vi "tb_interp_fft_fpga.vi"() -> ()   [LabVIEW 2011]
uses:
  <vilib>/Platform/TimedLoop/XDataNode/XDataNode.xnode
  <vilib>/Platform/TimedLoop/XDataNode/nitl_modes.ctl
  <vilib>/Platform/TimedLoop/XDataNode/XDNodeRunTimeDep.lvlib
  <vilib>/Platform/TimedLoop/XDataNode/wakeup.ctl
  <vilib>/Platform/TimedLoop/XDataNode/timing_clust.ctl
  <vilib>/rvi/DataTransferAndStorage/Container/XNode/niFpgaContainer.xnode
  <vilib>/rvi/FXPMathLib/FxpInterpret/XNode/nifxpmath_Interpret.xnode
  <userlib>/FPGA Library/Code Development/Signal Processing/Interpolation Block/Controls/Interpolation Input Data.ctl
  <vilib>/eio/EIONode/EIONode.xnode
  <vilib>/rvi/FIFO/Fifo_Resource/nirvififoEmulationGetNumberOfElementsToRead.vi
  <vilib>/rvi/FIFO/Fifo_Resource/nirvififoEmulationRead.vi
  <vilib>/rvi/interface/RandomDataEmulation/nirviRandomDataFpgaReadWriteTemplate.vi
  <vilib>/rvi/FIFO/Fifo_Resource/nirvififoEmulationWrite.vi
  <vilib>/rvi/eio/common/nirviEmuTemplateMethod_errors.vi
  <userlib>/FPGA Library/Code Development/Signal Processing/FFT Block/FFT/Controls/FFT States.ctl
  <userlib>/FPGA Library/Code Development/Signal Processing/FFT Block/FFT/Controls/FFT Parameters.ctl
panel:
  in  "FFT Parameters":T1={"Direction"=TRUE, "scale_sch"=85.0, "Flush Length"=0} {"scale_sch" format="%.0b"}
  in  "FFT State":cluster{"FFT State":T2, "Set FFT State?":bool}
  out "acq timed out?":bool
  out "Numeric":i32
  out "Interp Loop Overflow":bool
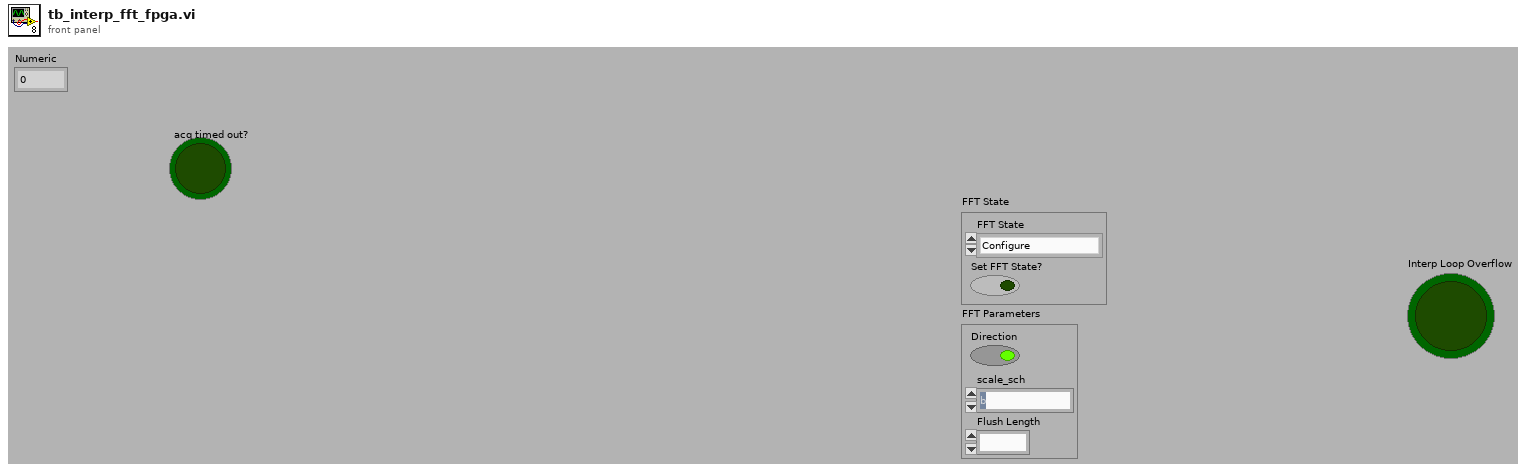
[diagram p1: front panel]
types:
  T1 = typedef "FFT Parameters.ctl" = cluster{"Direction":bool, "scale_sch":fxp<+,10,10>, "Flush Length":u16}
  T2 = typedef "FFT States.ctl" = enum8{"Configure", "Start FFT processing", "Process", "Unload Last FFT", "Reset"}
  T3 = typedef "XDNodeRunTimeDep.lvlib/timing_clust.ctl" = cluster{"Expected End [f-1]":u64, "Actual End [f-1]":u64, "Finished Late? [f-1]":bool, "Expected End [i-1]":u64, "Actual End [i-1]":u64, "Finished Late? [i-1]":bool, "Expected Start [i]":u64, "Actual Start [i]":u64, "Expected Start [f]":u64, "Actual Start [f]":u64, "Source Name":string, "Structure Name":string, "Period":i64, "Deadline":i64, "Offset":i64, "Start":i64, "Priority":i32, "Timeout":i32, "Mode":T4, "Wakeup Reason":T5, "Error":errorcluster, "Source Type":string, "Secondary Source Type":string, "Global End Time":u64, "Global Start Time":u64, "Frame Duration":u64, "Iteration Duration":u64, "Assigned CPU":i32, "I/O Scan Engine Mode":u32}
  T4 = typedef "XDNodeRunTimeDep.lvlib/nitl_modes.ctl" = enum32{"No Change", "Process missed periods, maintain original phase", "Discard missed periods, maintain original phase", "Process missed periods, ignore original phase", "Discard missed periods, ignore original phase"}
  T5 = typedef "XDNodeRunTimeDep.lvlib/wakeup.ctl" = enum32{"Normal", "Aborted", "Asynchronous wakeup", "Timing source error", "Timed loop error", "Timeout"}
  T6 = typedef "Interpolation Input Data.ctl" = fxp<+/-,18,1>
  T7 = typedef "Interpolation Output Data.ctl" = fxp<+/-,19,1>
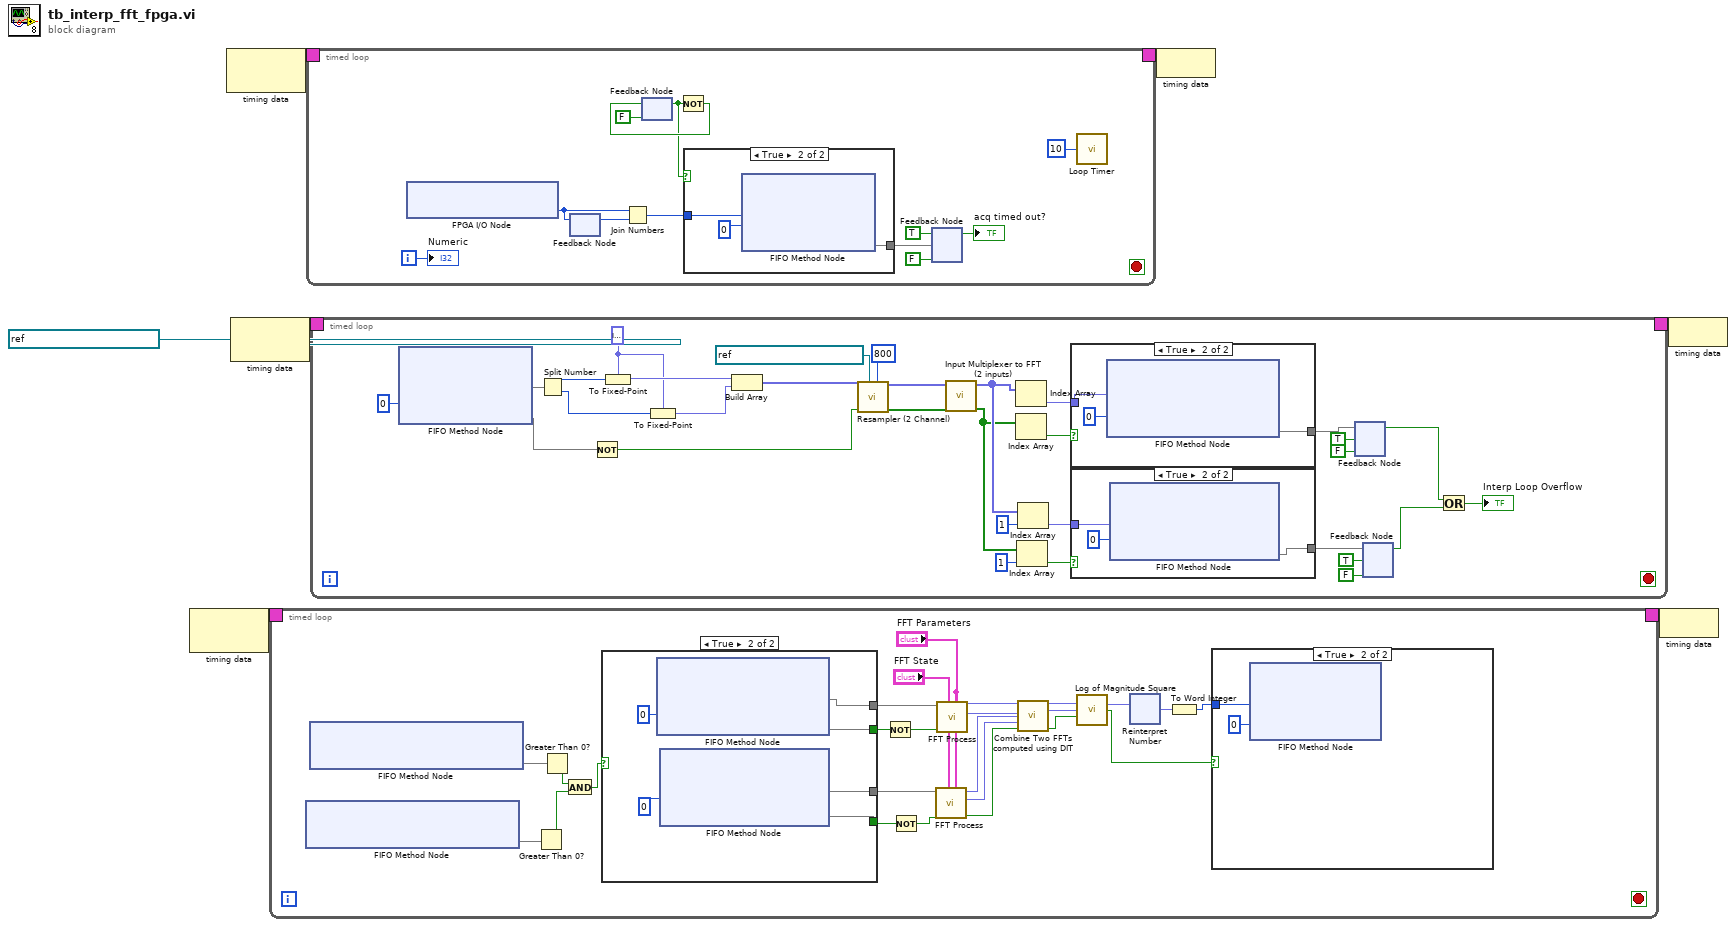
[diagram p0: block diagram]
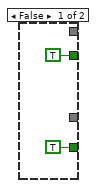
[diagram p4: hidden frame]
diagram:
  n1 = node-c288() -> (w5:T3)  [unwired: 1 in]
  n2 = node-c288() -> (w2:T3)  [unwired: 1 in]
  n3 = node-c288(refnum<k21> "40 MHz Onboard Clock" ("Source Name")) -> (w7:T3)
  n4 = timed-loop {
    timing: w5 -> [_]
    timing-out: [_] -> w4
    stop <- _ stop-if-true
    n5 = xnode ("FIFO Method Node")() -> ("Number of Elements to Read"=w24)  [unwired: 1 in, 1 out]
    n6 = xnode ("FIFO Method Node")() -> ("Number of Elements to Read"=w25)  [unwired: 1 in, 1 out]
    n7 = Greater Than 0?(x=w24) -> (x > 0?=w22:bool)
    n8 = Greater Than 0?(x=w25) -> (x > 0?=w23:bool)
    n9 = And(x=w23, y=w22) -> (x .and. y?=w21:bool)
    n10 = case shown="True" w21 {
      tunnel: [TRUE ("Timed Out?") w40] -> w32
      tunnel: [_ w39] -> w31
      tunnel: [_ w38] -> w30
      tunnel: [TRUE ("Timed Out?") w37] -> w29
      frame False {
      }
      frame True {
        n11 = xnode ("FIFO Method Node")("Timeout"=0) -> ("Element"=w39, "Timed Out?"=w40)  [unwired: 1 in, 1 out]
        n12 = xnode ("FIFO Method Node")("Timeout"=0) -> ("Element"=w38, "Timed Out?"=w37)  [unwired: 1 in, 1 out]
      }
    }
    n13 = Not(x=w32) -> (.not. x?=w26:bool)
    n14 = Not(x=w29) -> (.not. x?=w27:bool)
    n15 = call <userlib>:"FFT Process.vi"("FFT Parameters"="FFT Parameters", "FFT State"="FFT State", "Input Valid"=w27, "Real Data In"=w30) -> ("Output Valid"=w13:bool, "Imag Data Out"=w14:fxp<+/-,16,1>, "Real Data Out"=w15:fxp<+/-,16,1>)  [unwired: 2 in, 3 out]
    n16 = call <userlib>:"FFT Process.vi"("FFT Parameters"="FFT Parameters", "FFT State"="FFT State", "Input Valid"=w26, "Real Data In"=w31) -> ("Imag Data Out"=w16:fxp<+/-,16,1>, "Real Data Out"=w17:fxp<+/-,16,1>)  [unwired: 2 in, 4 out]
    n17 = call <userlib>:"Combine Two FFTs computed using DIT.vi"("Real FFT 1"=w17, "Imag FFT 1"=w16, "Real FFT 2"=w15, "Imag FFT 2"=w14, "Input Data Valid"=w13) -> ("Real FFT k"=w12:fxp<+/-,24,3>, "Imag FFT k"=w11:fxp<+/-,24,3>, "Output Valid"=w10:bool)  [unwired: 6 in, 2 out]
    n18 = call <userlib>:"Log of Magnitude Square.vi"("Real"=w12, "Imaginary"=w11, "Input Valid"=w10) -> ("Log Magnitude"=w20:fxp<+/-,34,12>, "Output Valid"=w18:bool)  [unwired: 11 in]
    n19 = xnode "Reinterpret Number"("x"=w20) -> ("y"=w28:fxp<+/-,34,16>)
    n20 = To Word Integer(number=w28) -> (16bit integer=w19:i16)
    n21 = case shown="True" w18 {
      tunnel: w19 -> [_ w34]
      frame False {
      }
      frame True {
        n22 = xnode ("FIFO Method Node")("Element"=w34, "Timeout"=0) -> ()  [unwired: 1 in, 2 out]
      }
    }
  }
  n23 = timed-loop {
    timing: w2 -> [_]
    timing-out: [_] -> w1
    i -> [w52]
    stop <- _ stop-if-true
    n24 = xnode "FPGA I/O Node"() -> ("IO Module\\AI 0 Data"=w61:i16)  [unwired: 1 in, 1 out]
    n25 = feedback-in #1(w61) -> ()
    n26 = feedback #1() -> (w60:i16)  [unwired: 1 in]
    n27 = Join Numbers(hi=w61, lo=w60) -> ((hi.lo)=w50:u32)
    n28 = feedback #2(FALSE) -> (w51:bool)
    n29 = Not(x=w51) -> (.not. x?=w59:bool)
    n30 = feedback-in #2(w59) -> ()
    n31 = case shown="True" w51 {
      tunnel: w50 -> [_ w64]
      tunnel: [_ w62] -> w55
      frame False {
      }
      frame True {
        n32 = xnode ("FIFO Method Node")("Element"=w64, "Timeout"=0) -> ("Timed Out?"=w62)  [unwired: 1 in, 1 out]
      }
    }
    n33 = feedback-in #3(TRUE, w55) -> ()
    n34 = feedback #3(FALSE) -> (→"acq timed out?":bool)
    n35 = call "Loop Timer"("Count(mSec)"=u32 10) -> ()  [unwired: 1 out]
    "Numeric" <- w52
  }
  n36 = timed-loop {
    timing: w7 -> [_]
    timing-out: [_] -> w6
    stop <- _ stop-if-true
    w72 = T6 0.0 ("Interpolate.Input Data")
    n37 = xnode ("FIFO Method Node")("Timeout"=0) -> ("Element"=w78, "Timed Out?"=w70)  [unwired: 1 in, 1 out]
    n38 = Split Number(x=w78) -> (hi(x)=w76:u16, lo(x)=w75:u16)
    n39 = Not(x=w70) -> (.not. x?=w69:bool)
    n40 = To Fixed-Point(fixed-point type=w72, number=w76) -> (fixed-point=w73:T6)
    n41 = To Fixed-Point(fixed-point type=w72, number=w75) -> (fixed-point=w74:T6)
    n42 = Build Array(w73, w74) -> (w71:T6[])
    n43 = call <userlib>:"Resampler (2 Channel).vi"("CalibrationTable Length-1"=u16 800, "ResampleVectorInfo"=refnum<k21> "Resample Vector Table", "DataValid"=w69, "Input Data"=w71) -> ("Data Valid"=w96:bool[], "Interpolated Data"=w97:T7[])  [unwired: 6 in]
    n44 = call <userlib>:"Input Multiplexer to FFT (2 inputs).vi"("Input Data Valid Array"=w96, "Input Data"=w97) -> ("Output Data Valid Array"=w91:bool[], "Interchanged Data"=w93:T7[])  [unwired: 8 in]
    n45 = Index Array(array=w93) -> (element=w95:T7)  [unwired: 1 in]
    n46 = Index Array(array=w91) -> (element=w94:bool)  [unwired: 1 in]
    n47 = Index Array(array=w91, index=1) -> (element=w90:bool)
    n48 = Index Array(array=w93, index=1) -> (element=w92:T7)
    n49 = case shown="True" w94 {
      tunnel: w95 -> [_ w103]
      tunnel: [_ w101] -> w87
      frame False {
      }
      frame True {
        n50 = xnode ("FIFO Method Node")("Element"=w103, "Timeout"=0) -> ("Timed Out?"=w101)  [unwired: 1 in, 1 out]
      }
    }
    n51 = case shown="True" w90 {
      tunnel: w92 -> [_ w100]
      tunnel: [_ w98] -> w84
      frame False {
      }
      frame True {
        n52 = xnode ("FIFO Method Node")("Element"=w100, "Timeout"=0) -> ("Timed Out?"=w98)  [unwired: 1 in, 1 out]
      }
    }
    n53 = feedback-in #4(w87, TRUE) -> ()
    n54 = feedback #4(FALSE ("Timed Out?")) -> (w83:bool)
    n55 = feedback #5(FALSE ("Timed Out?")) -> (w80:bool)
    n56 = feedback-in #5(w84, TRUE) -> ()
    n57 = Or(x=w83, y=w80) -> (x .or. y?=→"Interp Loop Overflow":bool)
  }
  n58 = node-c288(w1) -> ()
  n59 = node-c288(w4) -> ()
  n60 = node-c288(w6) -> ()
